vi "Set Tester Rx.vi"(8 "error in (no error)":errorcluster, 10 "ctl ref":refnum<vi>, 11 "Panel in":refnum<class "Panel.lvclass">) -> (0 "error out":errorcluster, 3 "Panel out":refnum<class "Panel.lvclass">)   [LabVIEW 2021, in "Panel.lvlib" / "Panel.lvclass"]
uses:
  Panel.lvclass
  Panel.lvclass/Panel.ctl
  <vilib>/OPCUA/server/Write Variant.vi
  <vilib>/OPCUA/NI OPC UA Server.lvlib
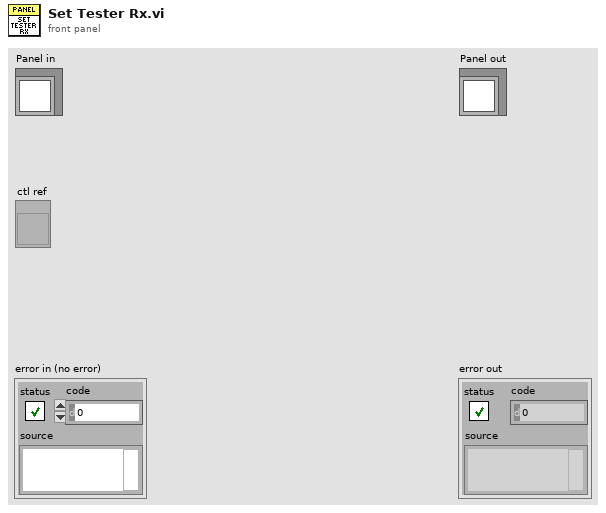
[diagram p1: front panel]
types:
  T1 = typedef "OPC UA Server Refnum.ctl" = refnum<k21>
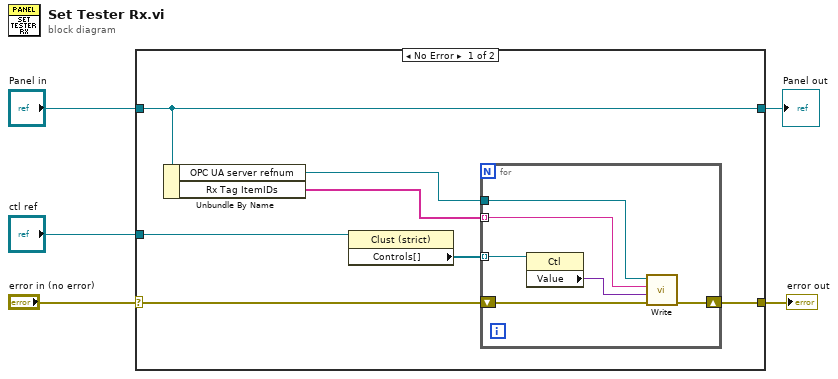
[diagram p0: block diagram]
diagram:
  n1 = case shown="No Error" "error in (no error)" {
    selector: "error in (no error)" -> [w7 w20]
    tunnel: [w6 w20] -> w4
    tunnel: [w12 w19] -> w2
    tunnel: "Panel in" -> [w12 w19]
    tunnel: "ctl ref" -> [w8 _]
    frame No Error {
      n2 = Unbundle By Name(w12) -> ("OPC UA server refnum"=w10:T1, "Rx Tag ItemIDs"=w9:string[])
      n3 = property class="Clust (strict)"(reference=w8) -> ("Controls[]"=w11:refnum<vi>[])  [unwired: 1 in, 2 out]
      n4 = for {
        tunnel: w10 -> [w18]
        tunnel: w9 -> [w16] mode=indexing
        tunnel: w11 -> [w15] mode=indexing
        shift-right: [w17] -> w6
        shift-left: w7 -> [w13]
        n5 = property class="Ctl"(reference=w15) -> ("Value"=w14:variant)  [unwired: 1 in, 2 out]
        n6 = call-poly <vilib>:"Write.vi"("error in (no error)"=w13, "value"=w14, "node ID"=w16, "OPC UA server refnum in"=w18) -> ("error out"=w17:errorcluster)  [unwired: 5 in, 2 out]
      }
    }
    frame Error {
    }
  }
  "error out" <- w4
  "Panel out" <- w2
